vi "ZAlign_RawAlignControls.vi"(8 "error in (no error)":errorcluster, 9 "Offset (Left and right)":i16, 10 "Refs":refnum<vi>[](array[refnum]), 11 "Panel in":refnum<vi>) -> (0 "error out":errorcluster, 2 "Positions":u32[](array[numeric]), 3 "Refs_Out":refnum<vi>[](array[refnum]))   [LabVIEW 2014, in "ZAlign.lvlib"]
doc: "ZAlign.lvlib:ZAlign_RawAlignControls.vi\n----------------------------------------------\nRaw Align controls\n\nInputs:\n---------------------\n- error in (no error) : Cluster; \n- Offset (Left and right) : I16; \n- Refs : 1DArrayOfRefnum; \n- Panel in : Refnum; \n\nOutputs:\n---------------------\n- error out : Cluster; \n- Positions : 1DArrayOfU32; \n- Refs_Out : 1DArrayOfRefnum; \n\n----------------------------------------------\n16/03/2015\nZühlke Engineering AG\nCH-8952 Schlieren\nwww.zuehlke.com"
uses:
  ZAlign.lvlib
panel:
  # "Connector Pane"
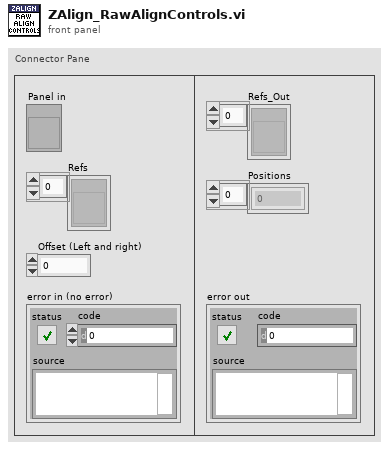
[diagram p1: front panel]
types:
  T1 = typedef "LVPositionTypeDef.ctl" = cluster{"Left":i32, "Top":i32}
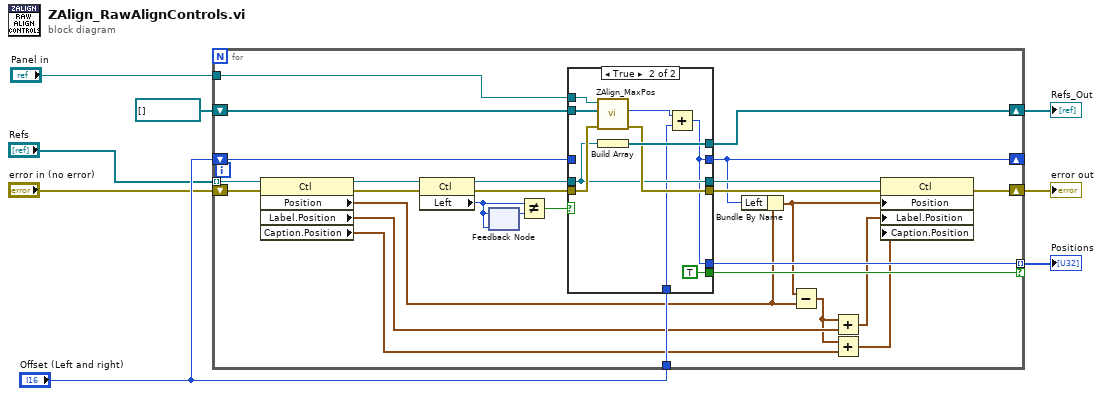
[diagram p0: block diagram]
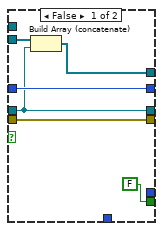
[diagram p2: hidden frame]
diagram:
  n1 = for {
    shift-right: [w34] -> w5
    shift-left: refnum<vi>[] [] -> [w33]
    shift-right: [w16] -> _
    shift-left: "Offset (Left and right)" -> [w30]
    tunnel: "Panel in" -> [w32]
    tunnel: "Refs" -> [w23] mode=indexing
    tunnel: [w27] -> w6 mode=indexing if=w26
    tunnel: "Offset (Left and right)" -> [w25]
    shift-right: [w19] -> w3
    shift-left: "error in (no error)" -> [w22]
    n2 = property class="Ctl"(reference=w23, error in=w22) -> (reference out=w20:refnum<vi>, error out=w21:errorcluster, "Position"=w12:T1, "Label.Position"=w15:T1, "Caption.Position"=w13:T1)
    n3 = property class="Ctl"(reference=w20, error in=w21) -> (reference out=w28:refnum<vi>, error out=w29:errorcluster, "Left"=w31:i32)
    n4 = feedback-in #1(w31) -> ()
    n5 = feedback #1(w31) -> (w35:i32)
    n6 = Not Equal?(x=w31, y=w35) -> (x != y?=w24:bool)
    n7 = case shown="True" w24 {
      tunnel: [w36 w51] -> w34
      tunnel: w33 -> [w41 w49]
      tunnel: [w40 w44] -> w16
      tunnel: w32 -> [_ w50]
      tunnel: w30 -> [w40 _]
      tunnel: [w39 w48] -> w18
      tunnel: w29 -> [w39 w47]
      tunnel: w28 -> [w38 w46]
      tunnel: [w38 w46] -> w17
      tunnel: [_ w44] -> w27
      tunnel: [FALSE TRUE] -> w26
      tunnel: w25 -> [_ w42]
      frame False {
        n8 = Build Array (concatenate)(w41, w38) -> (w36:refnum<vi>[])
      }
      frame True {
        n9 = call "ZAlign_MaxPos.vi"("error in (no error)"=w47, "Objects"=w49, "Panel"=w50) -> ("error out"=w48:errorcluster, "Max right location"=w45:u32)  [unwired: 6 in, 1 out]
        n10 = Build Array(w46) -> (w51:refnum<vi>[])
        n11 = Add(x=w45, y=w42) -> (x+y=w44:u32)
      }
    }
    n12 = Bundle By Name(cluster=w12, "Left"=w16) -> (w11:T1)
    n13 = Subtract(x=w11, y=w12) -> (x-y=w10:T1)
    n14 = Add(x=w10, y=w15) -> (x+y=w14:T1)
    n15 = Add(x=w10, y=w13) -> (x+y=w9:T1)
    n16 = property class="Ctl"(reference=w17, error in=w18, "Position"=w11, "Label.Position"=w14, "Caption.Position"=w9) -> (error out=w19:errorcluster)  [unwired: 1 out]
  }
  "Positions" <- w6
  "Refs_Out" <- w5
  "error out" <- w3
